vi "RODecode.vi"(11 "String":string) -> (0 "Current":dbl, 3 "Voltage":dbl)   [LabVIEW 2017]
panel:
  out "match substring 2":string
  out "match substring 3":string
  out "output cluster":T1
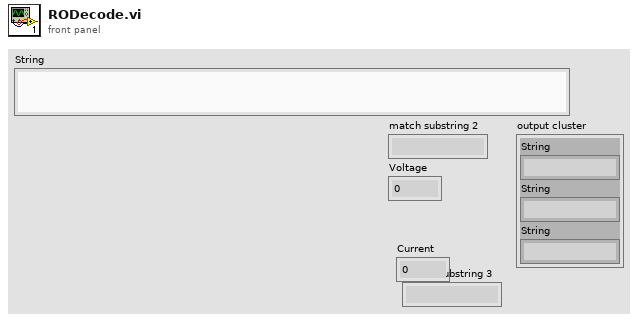
[diagram p1: front panel]
types:
  T1 = cluster{"String":string, "String":string, "String":string}
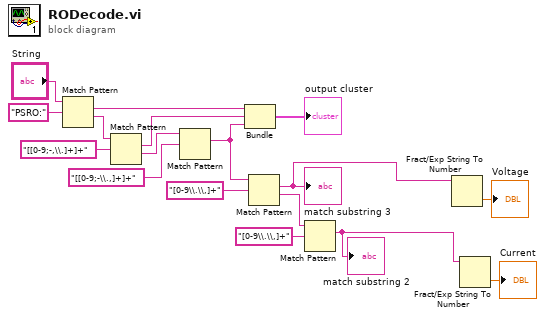
[diagram p0: block diagram]
diagram:
  n1 = Match Pattern(string="String", regular expression="PSRO:") -> (match substring=w11:string, after substring=w15:string)  [unwired: 1 in, 2 out]
  n2 = Match Pattern(string=w15, regular expression="[[0-9;-,\\.]+]+") -> (match substring=w10:string, after substring=w12:string)  [unwired: 1 in, 2 out]
  n3 = Match Pattern(string=w12, regular expression="[[0-9;-\\.,]+]+") -> (match substring=w8:string)  [unwired: 1 in, 3 out]
  n4 = Bundle("String"=w11, "String"=w10, "String"=w8) -> (→"output cluster":T1)  [unwired: 1 in]
  n5 = Match Pattern(string=w8, regular expression="[0-9\\.\\,]+") -> (match substring=w4:string, after substring=w6:string)  [unwired: 1 in, 2 out]
  "match substring 3" <- w4
  n6 = Match Pattern(string=w6, regular expression="[0-9\\.\\,]+") -> (match substring=w1:string)  [unwired: 1 in, 3 out]
  "match substring 2" <- w1
  n7 = Fract/Exp String To Number(string=w4) -> (number=→"Voltage":dbl)  [unwired: 3 in, 1 out]
  n8 = Fract/Exp String To Number(string=w1) -> (number=→"Current":dbl)  [unwired: 3 in, 1 out]
